vi "read_environment (SubVI).vi"(8 "data tasks":T1, 10 "Read pressures?":bool, 11 "Read temps?":bool) -> (0 "data tasks out":T1, 3 "environ cluster":cluster{dbl[], dbl[]})   [LabVIEW 2014]
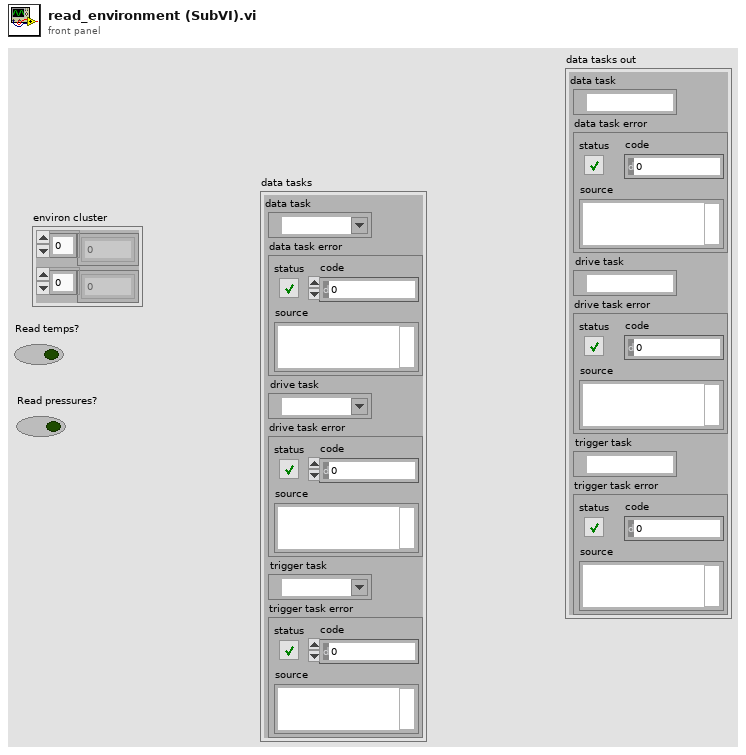
[diagram p1: front panel]
types:
  T1 = cluster{"data task":refnum<k21>, "data task error":errorcluster, "drive task":refnum<k21>, "drive task error":errorcluster, "trigger task":refnum<k21>, "trigger task error":errorcluster}
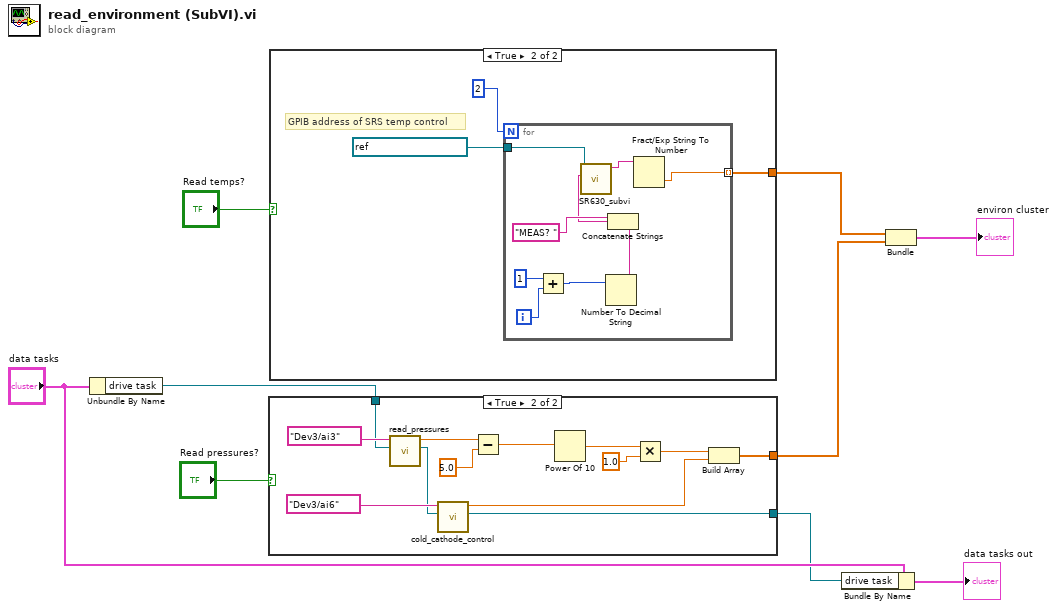
[diagram p0: block diagram]
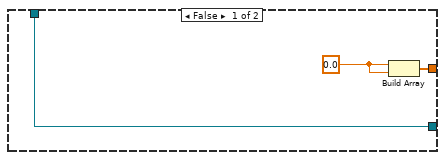
[diagram p2: hidden frame]
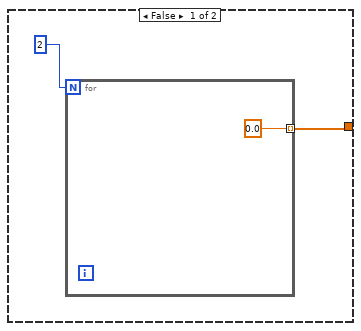
[diagram p3: hidden frame]
diagram:
  n1 = Unbundle By Name("data tasks") -> ("drive task"=w4:refnum<k21>)
  n2 = case shown="True" "Read pressures?" {
    tunnel: [w12 w16] -> w7
    tunnel: w4 -> [w10 w15]
    tunnel: [w10 w13] -> w2
    frame False {
      w11 = 0.0 ("element")
      n3 = Build Array(w11, w11) -> (w12:dbl[])
    }
    frame True {
      n4 = call "read_pressures.vi"("press task in"=w15, "Channel 1"=tag "Dev3/ai3") -> ("press task out"=w14:refnum<k21>, "Ch. 1 value"=w24:dbl)  [unwired: 8 in]
      n5 = call "cold_cathode_control.vi"("press task in"=w14, "Cold Cathode Gauge Channel"=tag "Dev3/ai6") -> ("press task out"=w13:refnum<k21>, "Cold Cathode Gauge Pressure"=w17:dbl)  [unwired: 8 in]
      n6 = Subtract(x=w24, y=5.0) -> (x-y=w23:dbl)
      n7 = Power Of 10(x=w23) -> (10^x=w22:dbl)
      n8 = Multiply(x=w22, y=1.0) -> (x*y=w18:dbl)
      n9 = Build Array(w18, w17) -> (w16:dbl[])
    }
  }
  n10 = case shown="True" "Read temps?" {
    tunnel: [w26 w29] -> w6
    frame False {
      n11 = for {
        N: 2 ("dimension size") -> [_]
        tunnel: [0.0] -> w26 mode=indexing
      }
    }
    frame True {
      # "GPIB address of SRS temp control"
      n12 = for {
        N: 2 ("dimension size") -> [_]
        tunnel: refnum<visa-resource-name> "GPIB0::19::INSTR" ("VISA Refnum in") -> [w40]
        tunnel: [w38] -> w29 mode=indexing
        i -> [w37]
        n13 = Add(x=1, y=w37) -> (x+y=w35:i32)
        n14 = Number To Decimal String(number=w35) -> (decimal integer string=w34:string)  [unwired: 1 in]
        n15 = Concatenate Strings("MEAS? " ("Write Buffer"), w34) -> (w32:string)
        n16 = call "SR630_subvi.vi"("Write Buffer"=w32, "VISA Refnum in"=w40) -> ("read buffer"=w39:string)  [unwired: 9 in]
        n17 = Fract/Exp String To Number(string=w39) -> (number=w38:dbl)  [unwired: 3 in, 1 out]
      }
    }
  }
  n18 = Bundle By Name(cluster="data tasks", "drive task"=w2) -> (→"data tasks out":T1)
  n19 = Bundle(w6, w7) -> (→"environ cluster":cluster{dbl[], dbl[]})  [unwired: 1 in]
